vi "Execute.vi"(8 "Error In":errorcluster, 9 "Workspace":T1, 10 "Control In":T2, 11 "Dispense in":refnum<class "Dispense.lvclass">) -> (0 "Error Out":errorcluster, 2 "Control Out":T2, 3 "Dispense in 2":refnum<class "Dispense.lvclass">)   [LabVIEW 2019, in "Dispense.lvclass"]
uses:
  Dispense.lvclass
  Controller/Controllers.ctl
  Controller/I-O/I-O.lvclass
  Controller/Dispenser/Dispenser.lvclass
  C:/Program Files (x86)/Aerotech/A3200/LabVIEW/2010/Bin/Aerotech.A3200.dll
  Program Files (x86)/Aerotech/A3200/LabVIEW/2010/Bin/Aerotech.A3200.dll
  Workspace/Workspace.ctl
  Dispense.lvclass/Dispense.ctl
  Controller/Motion/A3200/A3200.lvclass
  Controller/Controller.lvclass
  Workspace/Fixture.lvclass
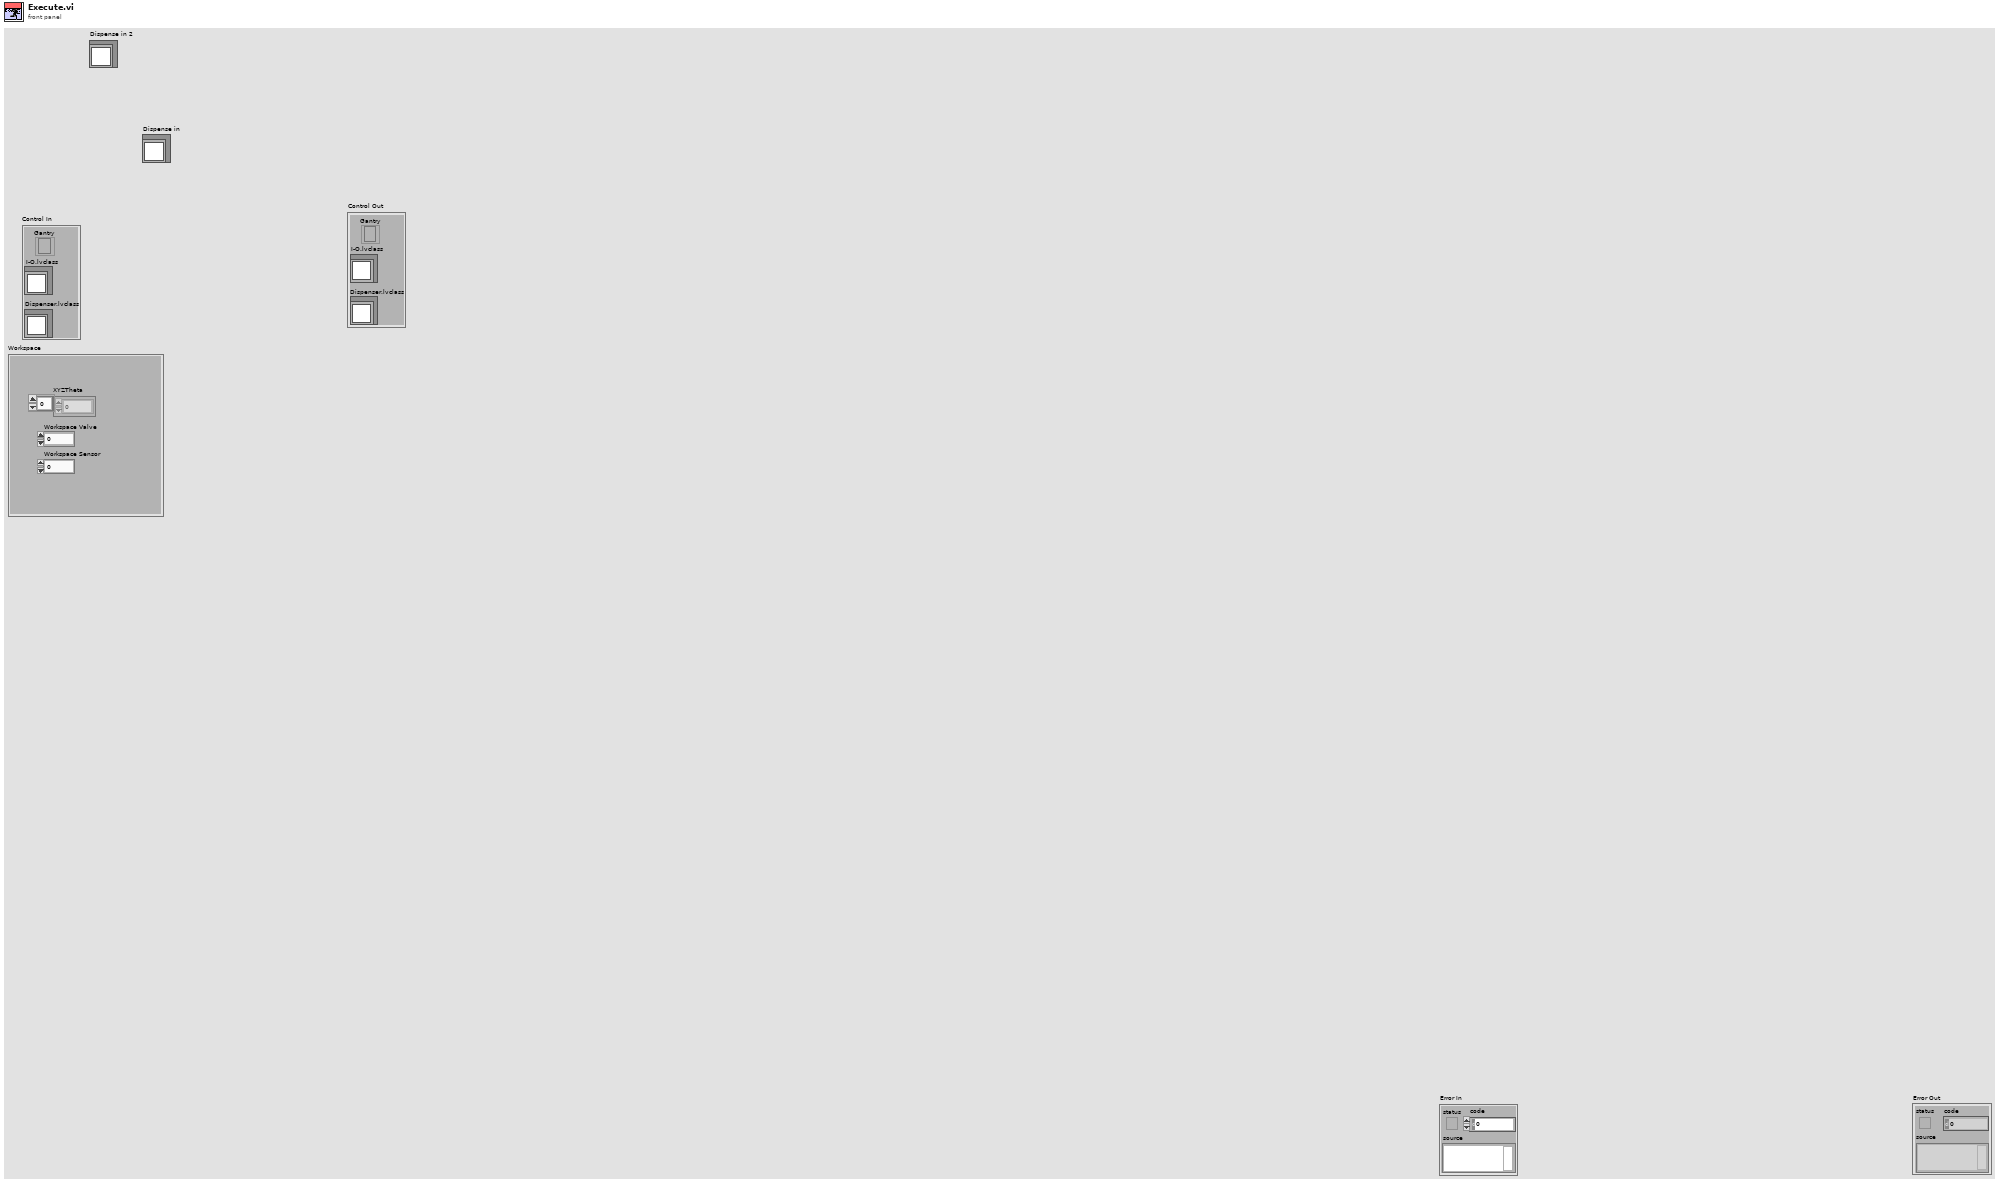
[diagram p1: front panel]
types:
  T1 = typedef "Fixture.lvclass/Workspace.ctl" = cluster{"XYZTheta":dbl[], "Workspace Valve":i32, "Workspace Sensor":i32}
  T2 = typedef "Controller.lvclass/Controllers.ctl" = cluster{"I-O.lvclass":refnum<class "I-O.lvclass">, "Dispenser.lvclass":refnum<class "Dispenser.lvclass">, "Gantry":refnum<k24>}
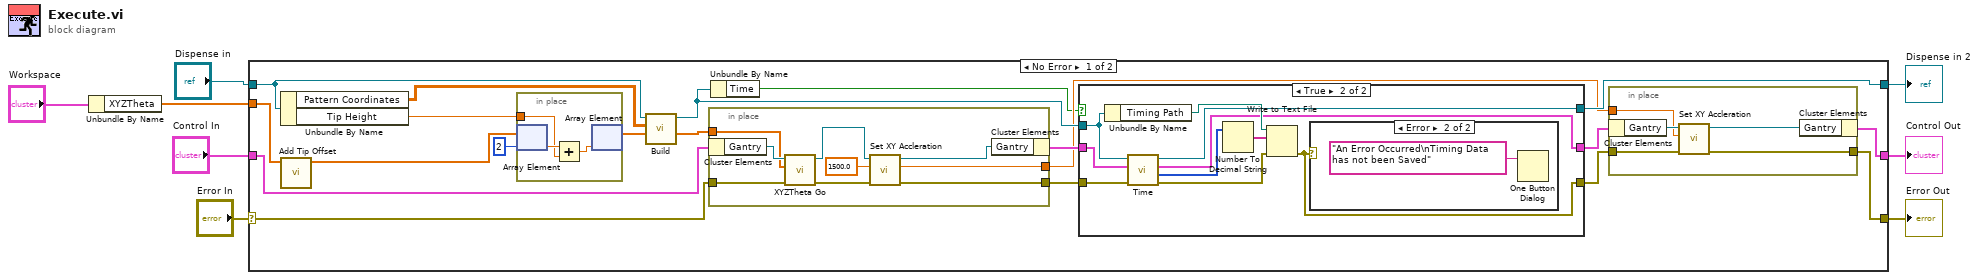
[diagram p0: block diagram]
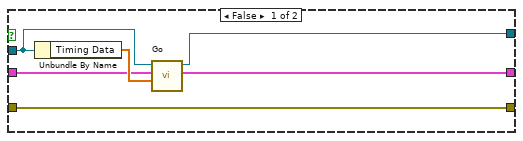
[diagram p2: hidden frame]
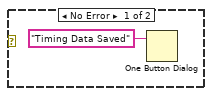
[diagram p3: hidden frame]
diagram:
  n1 = Unbundle By Name("Workspace") -> ("XYZTheta"=w2:dbl[])
  n2 = case shown="No Error" "Error In" {
    selector: "Error In" -> [w12 w65]
    tunnel: "Control In" -> [w21 w66]
    tunnel: [w15 w66] -> w7
    tunnel: "Dispense in" -> [w20 w64]
    tunnel: [w11 w65] -> w4
    tunnel: w2 -> [w19 _]
    tunnel: [w27 w64] -> w1
    frame No Error {
      n3 = Unbundle By Name(w20) -> ("Pattern Coordinates"=w25:dbl[][], "Tip Height"=w22:dbl)
      n4 = call "Add Tip Offset.vi"("XYZTheta"=w19) -> ("XYZTheta"=w18:dbl[])  [unwired: 10 in]
      n5 = in-place {
        in-place-border: w22 -> [w34]
        n6 = in-place-array #1(w18, 2) -> (w36:dbl)
        n7 = Add(x=w36, y=w34) -> (x+y=w35:dbl)
        n8 = in-place-array #1(w35) -> (w23:dbl[])  [unwired: 1 out]
      }
      n9 = call-dynamic "Build.vi"("XYZTheta"=w23, "Pattern Coordinates"=w25, "Dispense in"=w20) -> ("Starting Coordinates"=w26:dbl[], "Dispense out"=w28:refnum<class "Dispense.lvclass">)  [unwired: 7 in]
      n10 = in-place {
        in-place-border: w26 -> [w44]
        in-place-border: [w41] -> w14
        in-place-border: w12 -> [w39]
        in-place-border: [w37] -> w10
        n11 = in-place-cluster #2(w21) -> ("Gantry"=w45:refnum<k24>)
        n12 = call "XYZTheta Go.vi"("error in (no error)"=w39, "XYZTheta In"=w44, "Gantry In"=w45) -> ("error out"=w38:errorcluster, "Gantry Out"=w42:refnum<k24>)  [unwired: 6 in, 1 out]
        n13 = call "Set XY Accleration.vi"("Gantry In"=w42, "mm/s"=1500.0, "error in (no error)"=w38) -> ("Gantry Out"=w40:refnum<k24>, "X"=w41:dbl, "error out"=w37:errorcluster)  [unwired: 5 in]
        n14 = in-place-cluster #2("Gantry"=w40) -> (w17:T2)
      }
      n15 = Unbundle By Name(w28) -> ("Time"=w13:bool)
      n16 = case shown="True" w13 {
        tunnel: w28 -> [w48 w56]
        tunnel: w17 -> [w47 w58]
        tunnel: [w51 w57] -> w16
        tunnel: [w49 w55] -> w27
        tunnel: w10 -> [w46 w54]
        tunnel: [w46 w52] -> w9
        frame False {
          n17 = Unbundle By Name(w48) -> ("Timing Data"=w50:dbl[])
          n18 = call-dynamic "Go.vi"("Timing Data"=w50, "Control In"=w47, "Dispense in"=w48) -> ("Control Out"=w51:T2, "Dispense Out"=w49:refnum<class "Dispense.lvclass">)  [unwired: 7 in]
        }
        frame True {
          n19 = Unbundle By Name(w56) -> ("Timing Path"=w60:path)
          n20 = call-dynamic "Time.vi"("error in (no error)"=w54, "Control In"=w58, "Dispense in"=w56) -> ("error out"=w53:errorcluster, "Timing Data"=w59:i32[], "Control Out"=w57:T2, "Dispense out"=w55:refnum<class "Dispense.lvclass">)  [unwired: 5 in]
          n21 = Number To Decimal String(number=w59) -> (decimal integer string=w61:string[])  [unwired: 1 in]
          n22 = Write to Text File(file (use dialog)=w60, text=w61, error in=w53) -> (error out=w52:errorcluster)  [unwired: 1 in, 2 out]
          n23 = case shown="Error" w52 {
            frame No Error {
              n24 = One Button Dialog(message="Timing Data Saved") -> ()  [unwired: 1 in, 1 out]
            }
            frame Error {
              n25 = One Button Dialog(message="An Error Occurred\nTiming Data has not been Saved") -> ()  [unwired: 1 in, 1 out]
            }
          }
        }
      }
      n26 = in-place {
        in-place-border: w14 -> [w31]
        in-place-border: w9 -> [w30]
        in-place-border: [w29] -> w11
        n27 = in-place-cluster #3(w16) -> ("Gantry"=w33:refnum<k24>)
        n28 = call "Set XY Accleration.vi"("Gantry In"=w33, "mm/s"=w31, "error in (no error)"=w30) -> ("Gantry Out"=w32:refnum<k24>, "error out"=w29:errorcluster)  [unwired: 5 in, 1 out]
        n29 = in-place-cluster #3("Gantry"=w32) -> (w15:T2)
      }
    }
    frame Error {
    }
  }
  "Control Out" <- w7
  "Error Out" <- w4
  "Dispense in 2" <- w1
